vi "SendSerialCommand.vi"(8 "error  in":errorcluster, 9 "Expected Response":string, 10 "Command":string, 11 "FPGA VI Reference In":refnum<k20>) -> (0 "error out":errorcluster, 3 "FPGA VI Reference out":refnum<k20>)   [LabVIEW 2010]
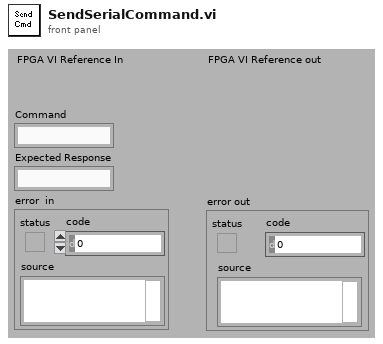
[diagram p1: front panel]
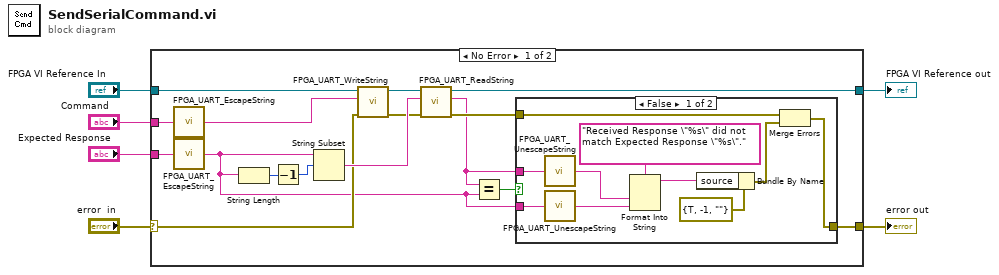
[diagram p0: block diagram]
diagram:
  n1 = case shown="No Error" "error  in" {
    selector: "error  in" -> [w11 w35]
    tunnel: "FPGA VI Reference In" -> [w22 w34]
    tunnel: [w20 w34] -> w5
    tunnel: "Command" -> [w10 _]
    tunnel: [w13 w35] -> w3
    tunnel: "Expected Response" -> [w8 _]
    frame No Error {
      n2 = call "FPGA_UART_EscapeString.vi"("Unescaped String"=w10) -> ("Escaped String"=w9:string)
      n3 = call "FPGA_UART_EscapeString.vi"("Unescaped String"=w8) -> ("Escaped String"=w7:string)
      n4 = String Length(string=w7) -> (length=w19:i32)
      n5 = Decrement(x=w19) -> (x-1=w18:i32)
      n6 = String Subset(string=w7, offset (0)=w18) -> (substring=w17:string)  [unwired: 1 in]
      n7 = call "FPGA_UART_WriteString.vi"("error  in"=w11, "String"=w9, "FPGA VI Reference In"=w22) -> ("error out"=w16:errorcluster, "FPGA UART Reference"=w21:refnum<k20>)  [unwired: 7 in]
      n8 = call "FPGA_UART_ReadString.vi"("error in"=w16, "TermChar"=w17, "FPGA VI Reference in"=w21) -> ("error out"=w14:errorcluster, "String"=w12:string, "FPGA VI Reference out"=w20:refnum<k20>)  [unwired: 6 in]
      n9 = Equal?(x=w12, y=w7) -> (x = y?=w15:bool)
      n10 = case shown="False" w15 {
        tunnel: w14 -> [w32 w33]
        tunnel: [w27 w33] -> w13
        tunnel: w7 -> [w24 _]
        tunnel: w12 -> [w26 _]
        frame False {
          n11 = call "FPGA_UART_UnescapeString.vi"("Escaped String"=w26) -> ("Unescaped String"=w25:string)
          n12 = call "FPGA_UART_UnescapeString.vi"("Escaped String"=w24) -> ("Unescaped String"=w23:string)
          n13 = Format Into String(format string="Received Response \"%s\" did not match Expected Response \"%s\".", w25, w23) -> (resulting string=w28:string)  [unwired: 2 in, 1 out]
          n14 = Bundle By Name(cluster=errorcluster {"status"=TRUE, "code"=-1, "source"=""} ("error out"), "source"=w28) -> (w29:errorcluster)
          n15 = Merge Errors(w32, w29) -> (w27:errorcluster)
        }
        frame True {
        }
      }
    }
    frame Error {
    }
  }
  "FPGA VI Reference out" <- w5
  "error out" <- w3
